vi "OPC DA client read.vi"() -> ()   [LabVIEW 2023]
panel:
  in  "Tab Control":enum32{"Options"}(tab)
  in  "OPC Tag":string="opc://localhost/Matrikon.OPC.Simulation.1/Bucket Brigade.Real4"
  in  "Select different OPC Tag":bool
  out "Temperature Chart":dbl(graph)
  out "Temperature":dbl format="%#_4g"
  in  "stop":bool
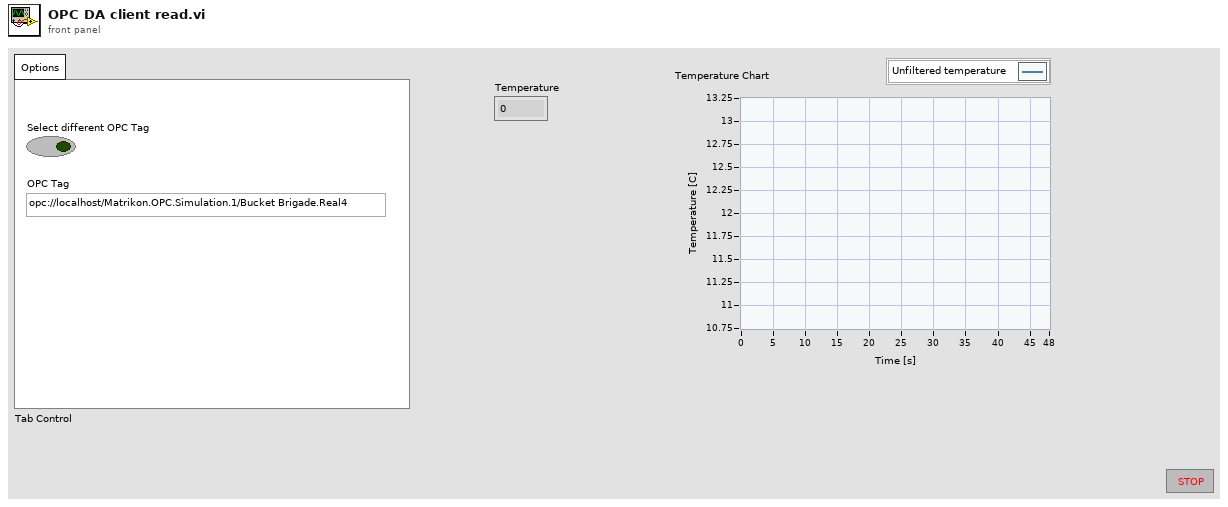
[diagram p1: front panel]
types:
  T1 = enum16{"Read", "Write", "ReadWrite", "BufferedRead", "BufferedReadWrite"}
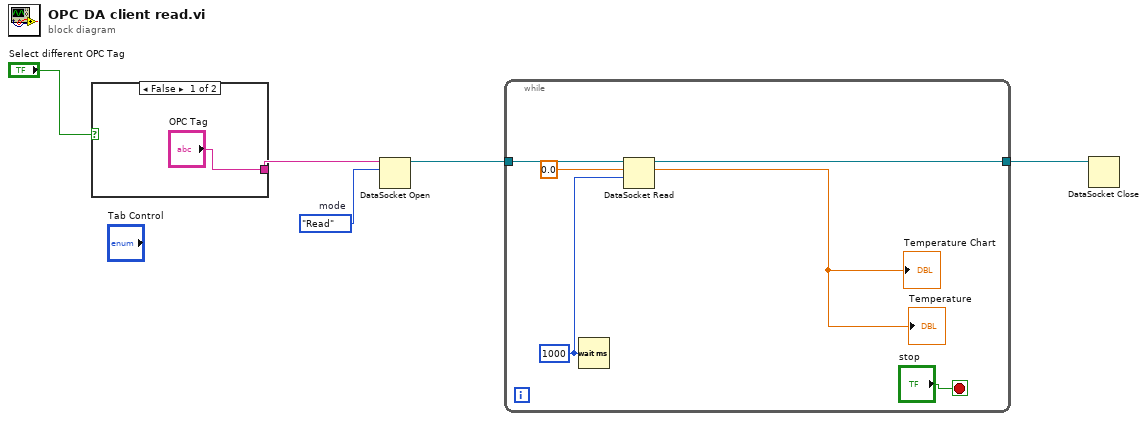
[diagram p0: block diagram]
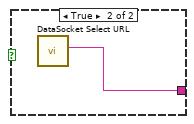
[diagram p2: hidden frame]
diagram:
  w5 = T1."Read"  # mode
  n1 = case shown="False" "Select different OPC Tag" {
    tunnel: ["OPC Tag" w7] -> w2
    frame False {
    }
    frame True {
      n2 = call <vilib>:"DataSocket Select URL.vi"() -> ("URL"=w7:string)  [unwired: 9 in, 2 out]
    }
  }
  n3 = DataSocket Open(10:w5, 11:w2) -> (3:w4:refnum<k13>)  [unwired: 2 in, 1 out]
  n4 = while {
    tunnel: w4 -> [w13]
    tunnel: [w12] -> w3
    stop <- "stop" stop-if-true
    w8 = u32 1000 ("milliseconds to wait")
    n5 = Wait (ms)(milliseconds to wait=w8) -> ()  [unwired: 1 out]
    n6 = DataSocket Read(9:w8, 10:0.0, 11:w13) -> (2:→"Temperature" →"Temperature Chart":dbl, 3:w12:refnum<k13>)  [unwired: 2 in, 5 out]
  }
  n7 = DataSocket Close(11:w3) -> ()  [unwired: 2 in, 2 out]
